vi "Write Thermocouple Diff Measured.vi"(10 "Thermocouple Diff Measured":dbl[unit] format="%.1f", 11 "Thermocouple in":refnum<class "Thermocouple.lvclass">) -> (3 "Thermocouple out":refnum<class "Thermocouple.lvclass">)   [LabVIEW 2013, in "Thermocouple.lvclass"]
uses:
  Thermocouple.lvclass
  Thermocouple.lvclass/Thermocouple.ctl
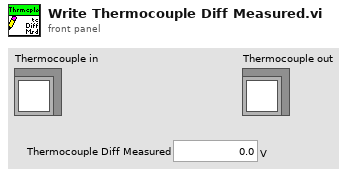
[diagram p1: front panel]
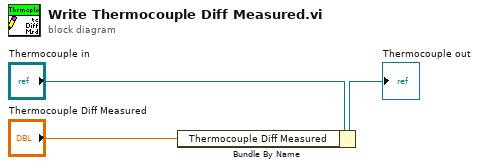
[diagram p0: block diagram]
diagram:
  n1 = Bundle By Name(cluster="Thermocouple in", "Thermocouple Diff Measured"="Thermocouple Diff Measured") -> (→"Thermocouple out":refnum<class "Thermocouple.lvclass">)
